vi "Status Instrument.vi"(0 "VISA resource name":refnum<visa-resource-name>, 11 "error in (no error)":errorcluster) -> (2 "Remote Interface Mode":u16(ring) items=["Local", "Remote", "Remote w/ Lockout"], 3 "Beeper Enabled/Disabled":bool, 4 "VISA resource name out":refnum<visa-resource-name>, 8 "Keypad Status":bool, 10 "Lock-Out":bool, 14 "Lock-Out Code":dbl min=0.0 max=999.0 step=1.0, 15 "error out":errorcluster)   [LabVIEW 2013, in "Lake Shore Cryotronics 331.lvlib"]
doc: "This VI displays various instrument settings. Parameters indicated are;\nRemote interface status\nKeypad lock-out status\nAudible beeper status\nKeypad status"
uses:
  Lake Shore Cryotronics 331.lvlib
panel:
  # "Keypad Lock-Out"
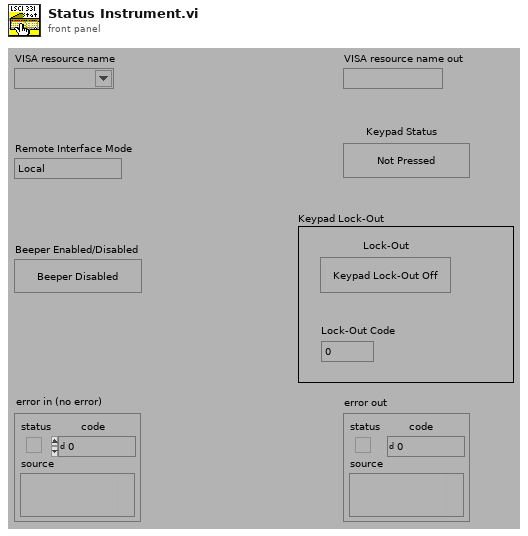
[diagram p1: front panel]
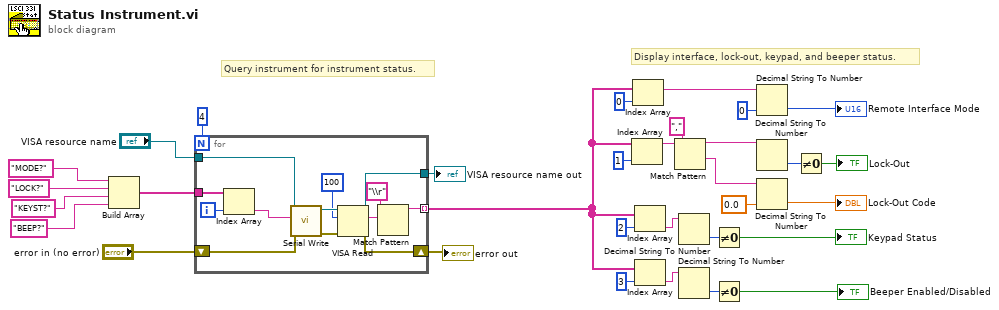
[diagram p0: block diagram]
diagram:
  # "Display interface, lock-out, keypad, and beeper status."
  # "Query instrument for instrument status."
  n1 = Build Array("MODE?", "LOCK?", "KEYST?", "BEEP?") -> (w27:string[])
  n2 = for {
    N: 4 -> [_]
    tunnel: w27 -> [w34]
    shift-right: [w39] -> w31
    shift-left: "error in (no error)" -> [w40]
    tunnel: [w38] -> w32
    tunnel: "VISA resource name" -> [w37]
    tunnel: [w35] -> w2 mode=indexing
    i -> [w41]
    n3 = Index Array(array=w34, index=w41) -> (element=w33:string)
    n4 = call "Serial Write.vi"("error in (no error)"=w40, "Write Buffer (\"\")"=w33, "VISA resource name"=w37) -> ("error out"=w44:errorcluster, "VISA resource name out"=w45:refnum<visa-resource-name>)  [unwired: 6 in, 1 out]
    n5 = VISA Read(VISA resource name=w45, byte count=100, error in (no error)=w44) -> (VISA resource name out=w38:refnum<visa-resource-name>, read buffer=w42:string, error out=w39:errorcluster)  [unwired: 1 out]
    n6 = Match Pattern(string=w42, regular expression="\\r") -> (before substring=w35:string)  [unwired: 1 in, 3 out]
  }
  "VISA resource name out" <- w32
  "error out" <- w31
  n7 = Index Array(array=w2, index=1) -> (element=w14:string)
  n8 = Index Array(array=w2, index=0) -> (element=w12:string)
  n9 = Index Array(array=w2, index=2) -> (element=w21:string)
  n10 = Index Array(array=w2, index=3) -> (element=w8:string)
  n11 = Match Pattern(string=w14, regular expression=",") -> (before substring=w15:string, after substring=w16:string)  [unwired: 1 in, 2 out]
  n12 = Decimal String To Number(string=w21) -> (number=w22:i32)  [unwired: 2 in, 1 out]
  n13 = Decimal String To Number(string=w8) -> (number=w7:i32)  [unwired: 2 in, 1 out]
  n14 = Not Equal To 0?(x=w22) -> (x != 0?=→"Keypad Status":bool)
  n15 = Not Equal To 0?(x=w7) -> (x != 0?=→"Beeper Enabled/Disabled":bool)
  n16 = Decimal String To Number(string=w12, default (0L)=u16 0) -> (number=→"Remote Interface Mode":u16)  [unwired: 1 in, 1 out]
  n17 = Decimal String To Number(string=w15) -> (number=w17:i32)  [unwired: 2 in, 1 out]
  n18 = Decimal String To Number(string=w16, default (0L)=0.0) -> (number=→"Lock-Out Code":dbl)  [unwired: 1 in, 1 out]
  n19 = Not Equal To 0?(x=w17) -> (x != 0?=→"Lock-Out":bool)
